vi "testbench.vi"() -> ()   [LabVIEW 2018]
panel:
  out "output":i32
  out "bitstream":i32[](array[numeric])
  in  "bits":i32
  in  "decimal":i32
  # "TESTBENCH"
  # "将十进制数decimal，\n转换为bits位的二进制数组bitstream"
  # "将二进制数组bitstream\n转换为十进制数output"
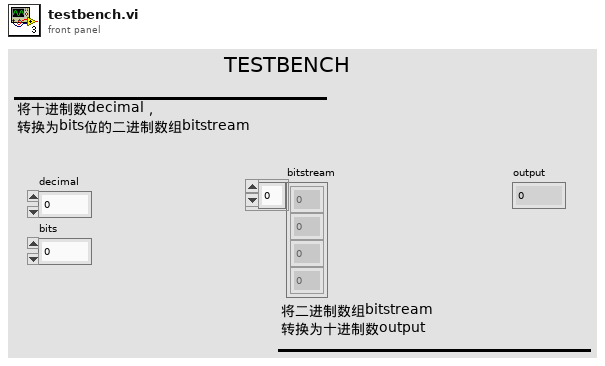
[diagram p1: front panel]
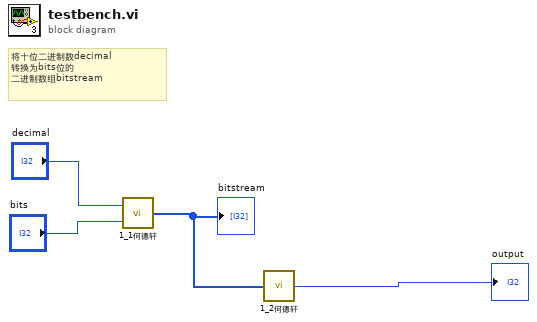
[diagram p0: block diagram]
diagram:
  # "将十位二进制数decimal\n转换为bits位的\n二进制数组bitstream"
  n1 = call "1_1何德轩.vi"("bits"="bits", "decimal"="decimal") -> ("bitstream"=w2:i32[])
  "bitstream" <- w2
  n2 = call "1_2何德轩.vi"("bitstream"=w2) -> ("output"=→"output":i32)
